vi "QX Thread.vi"() -> ()   [LabVIEW 2016]
uses:
  <vilib>/Utility/error.llb/DialogType.ctl
  Controls/hwSettings command.ctl
  DAQ-Display/Controls/PSDAQEG_Commoand Type.ctl
  DAQ-Display/PanelSplitToolkit/QueueManager.llb/CreatQueue.vi
  DAQ-Display/PanelSplitToolkit/QueueManager.llb/Remove.vi
  DAQ-Display/PanelSplitToolkit/QueueManager.llb/Insert.vi
  DAQ-Display/PanelSplitToolkit/QueueManager.llb/Destroy.vi
  DAQ-Display/PanelSplitToolkit/QueueManager.llb/Valid?.vi
panel:
  out "Waveform Chart":waveform(dbl)[](graph)
  out "Connect?":bool
  in  "Disconnect":bool
  in  "StopDAQ":bool
  in  "StartDAQ":bool
  in  "GetInfo":bool
  in  "Connect":bool
  in  "Caller":string
  # "QX硬件线程"
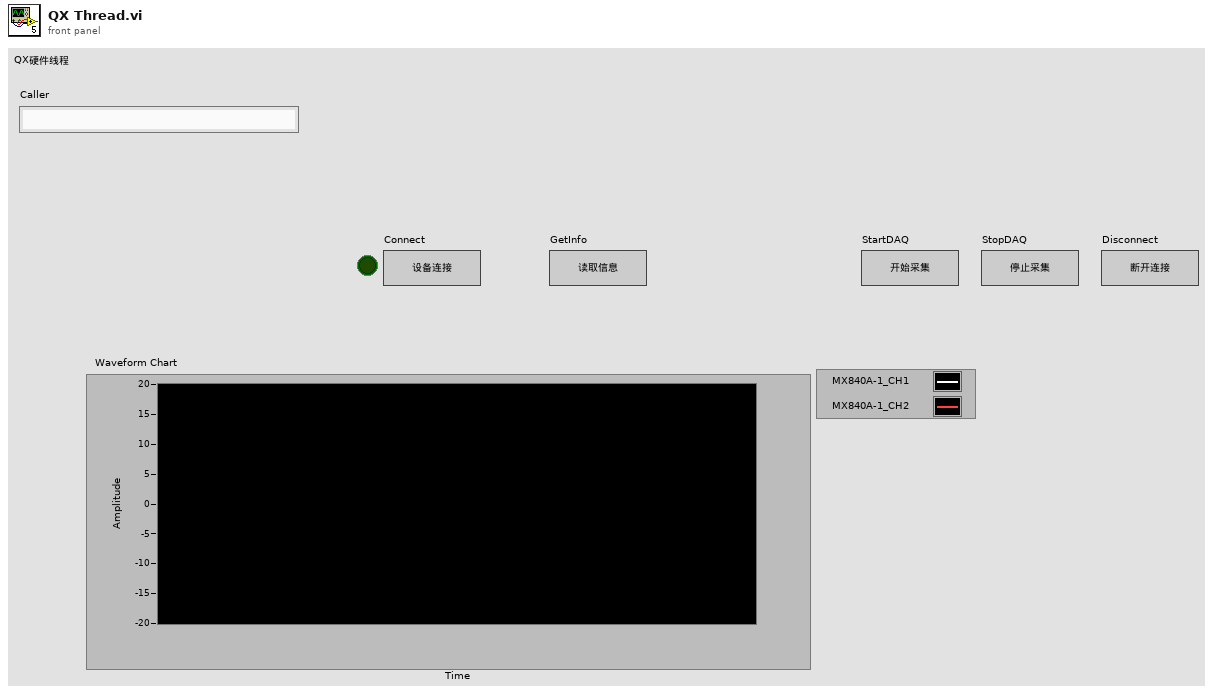
[diagram p1: front panel]
types:
  T1 = cluster{"Main Queue":string, "DAQ Queue":string, "ANA Queue":string, "CUI Queue":string, "Q-FocusList":string, "Q-Toolbar":string, "Q-Config":string}
  T2 = typedef "PSCHN_Channel Para.ctl" = cluster{"CHTag*":string, "Used?*":bool, "CHName":string, "Unit":string, "斜率":dbl, "截距":dbl}
  T3 = typedef "PSCHN_Card Para.ctl" = cluster{"Module Type":string, "Module Name":string, "ModuSN":string, "ModuIP":string, "Used?":bool, "Connected":bool, "Timing*":cluster{"Sample Rate":dbl}, "Channels":T2[]}
  T4 = typedef "hw_QX_hwDriverRef.ctl" = cluster{"DevicesAndSignals":cluster{"Devices":refnum<k24>[], "Signals":refnum<k24>[]}, "DaqMeasurement":refnum<k24>}
  T5 = cluster{"error":errorcluster, "LocalQ":cluster{"LQName":string, "LQEvent":string, "LQData":variant}, "HighQ":cluster{"HQName":string, "HQEvent":string, "HQData":variant}, "Channel":T2, "Card":T3, "hwType":string, "hwDriverRef":T4, "DevsInfo":T3[], "DataQ":string, "tdms ref":refnum<k34>, "Save":bool, "T0":timestamp}
  T6 = typedef "hwSettings command.ctl" = enum16{"Init", "Read", "Clear"}
  T7 = typedef "PSDAQEG_Commoand Type.ctl" = enum16{"Config", "Run", "Pause", "Stop", "Save", "Connect"}
  T8 = typedef "DialogType.ctl" = u16
  T9 = typedef "hwDefaultSetting.ctl" = cluster{"hwType":string, "hwNumber":u32, "hwName":string[], "hwSN":string[], "hwCHNumber":u32[]}
  T10 = cluster{string, string[], "Object Name":string}[]
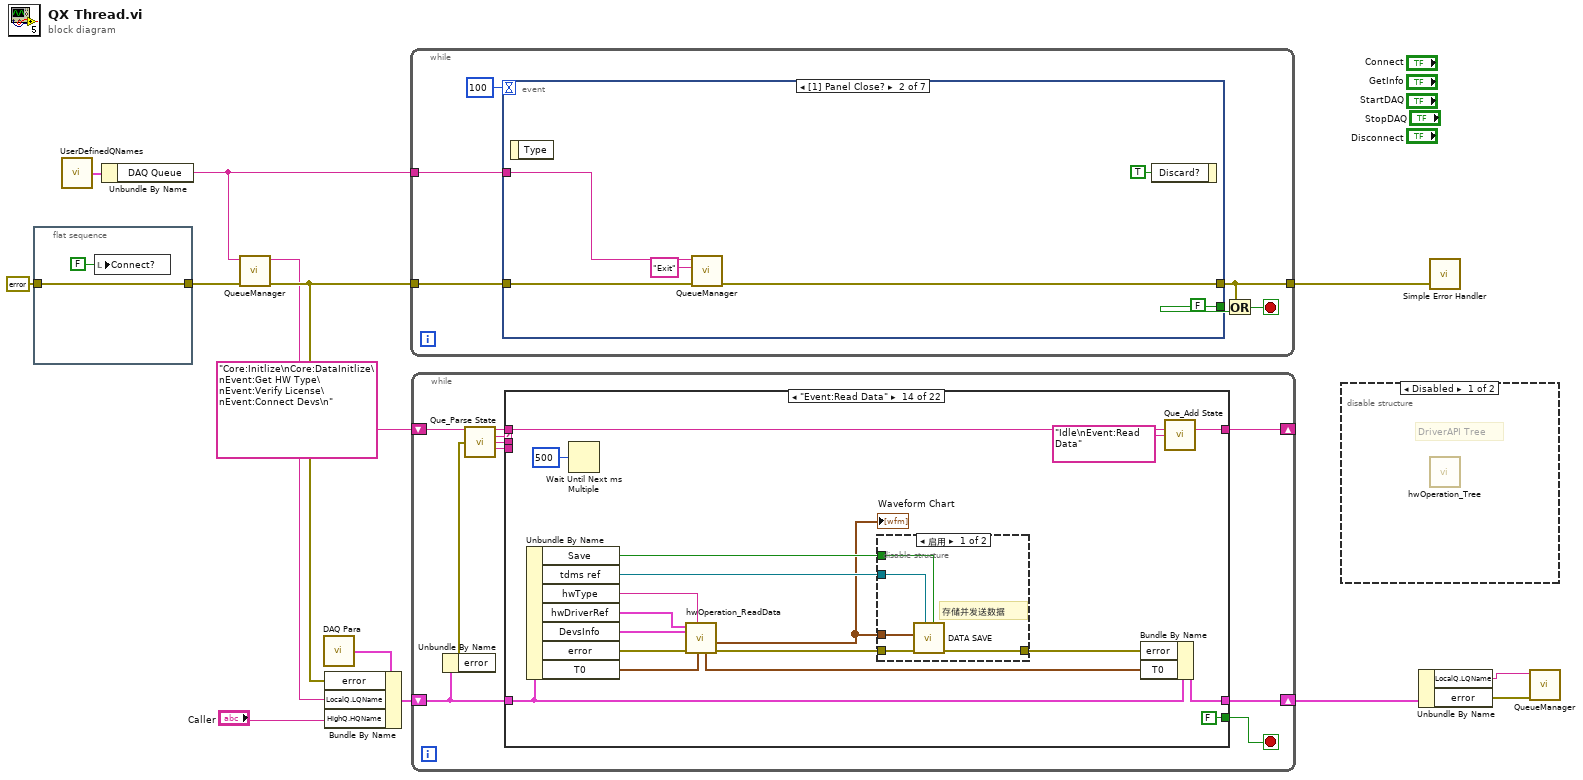
[diagram p0: block diagram]
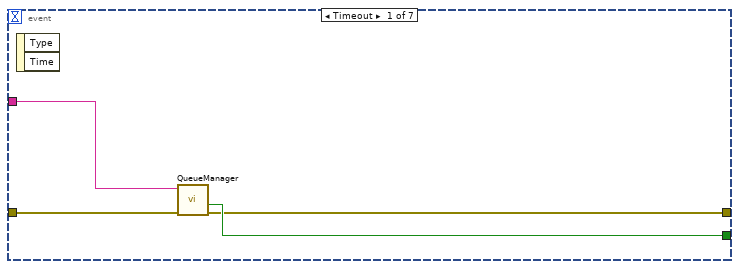
[diagram p3: hidden frame]
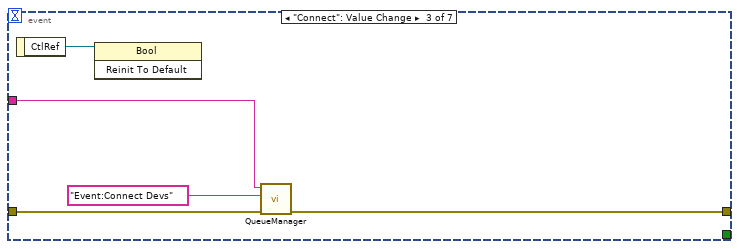
[diagram p4: hidden frame]
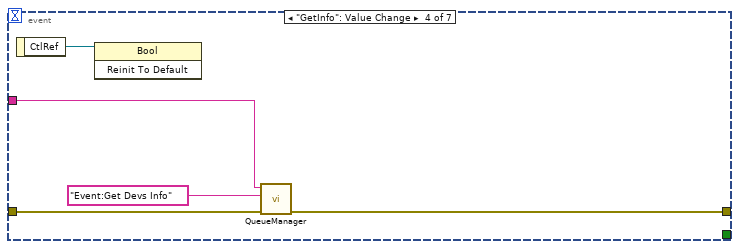
[diagram p5: hidden frame]
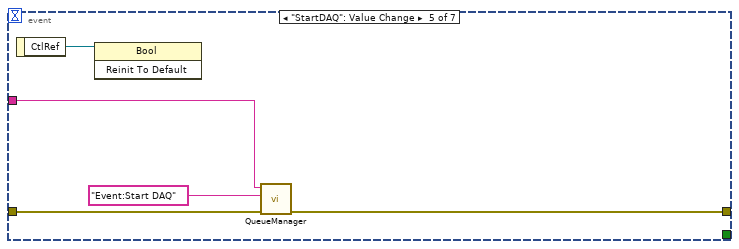
[diagram p6: hidden frame]
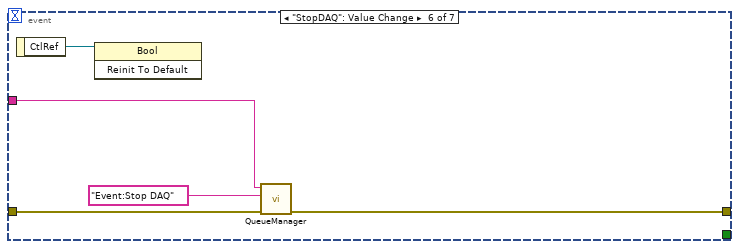
[diagram p7: hidden frame]
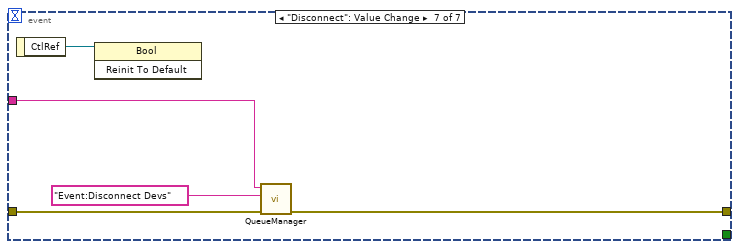
[diagram p8: hidden frame]
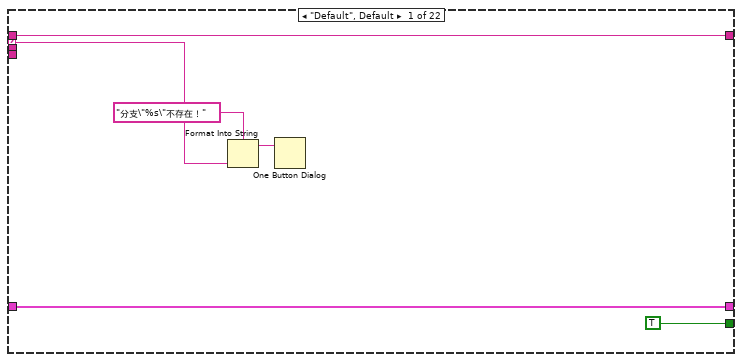
[diagram p9: hidden frame]
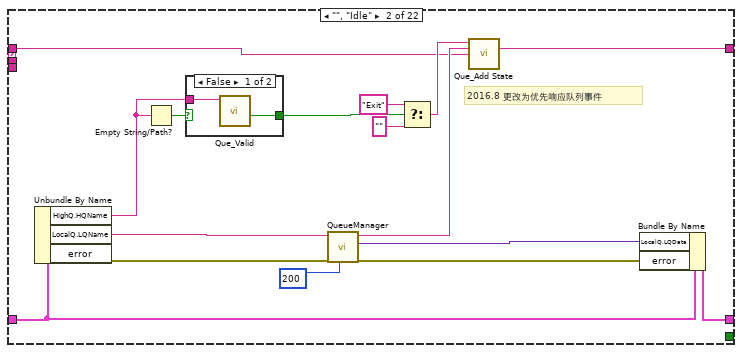
[diagram p10: hidden frame]
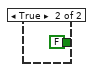
[diagram p11: hidden frame]
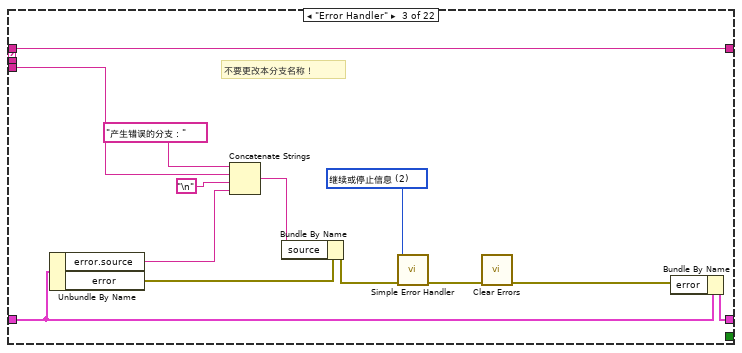
[diagram p12: hidden frame]
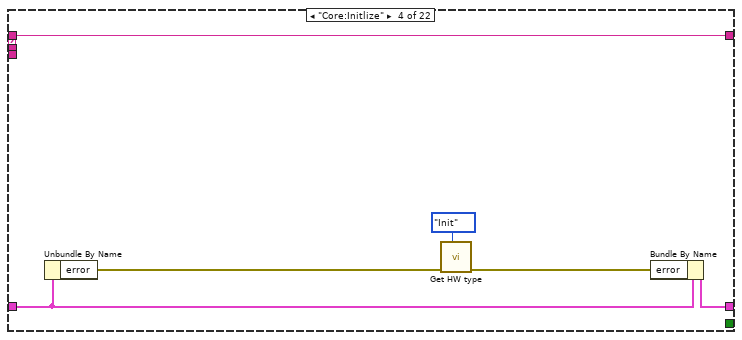
[diagram p13: hidden frame]
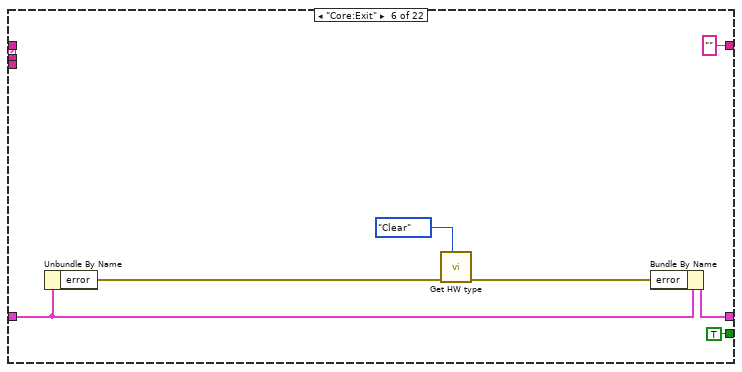
[diagram p15: hidden frame]
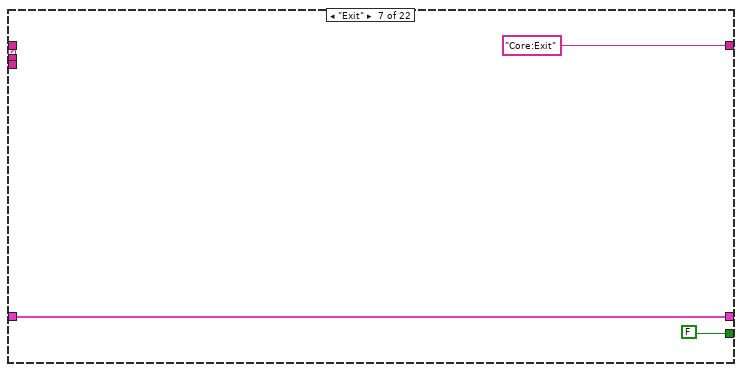
[diagram p16: hidden frame]
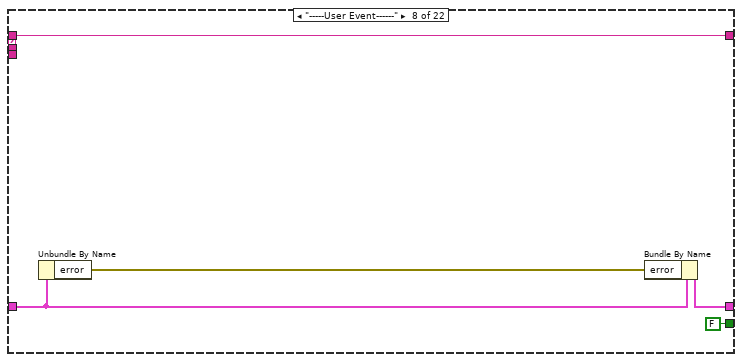
[diagram p17: hidden frame]
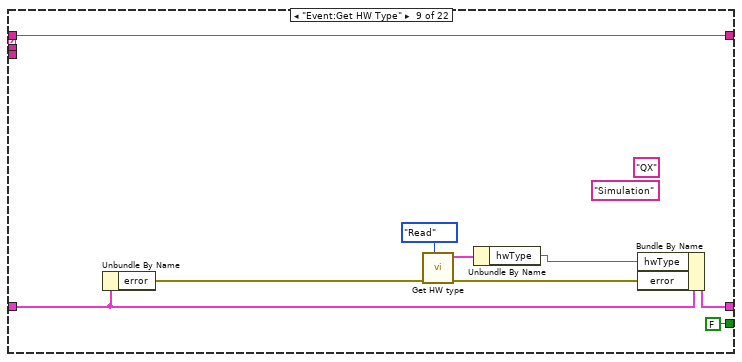
[diagram p18: hidden frame]
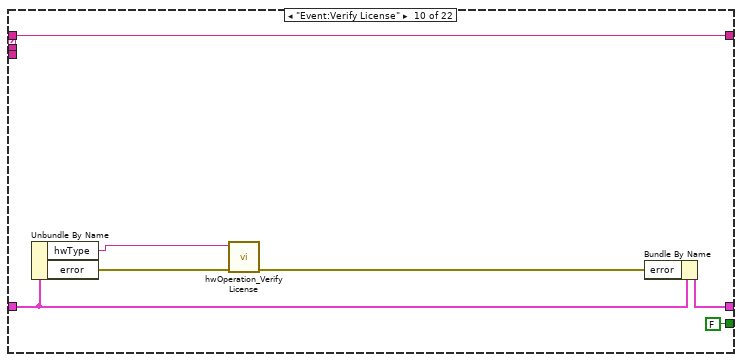
[diagram p19: hidden frame]
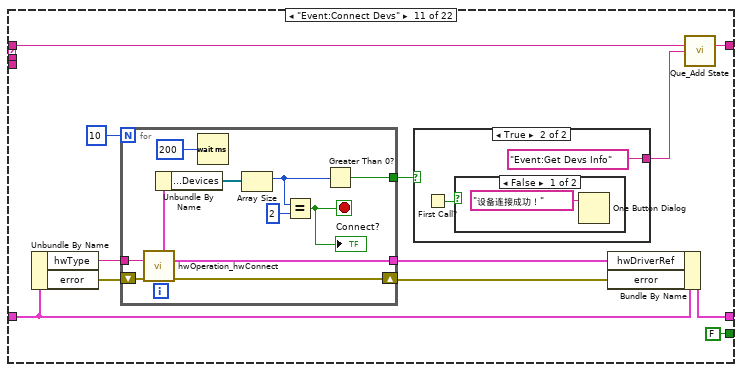
[diagram p20: hidden frame]
diagram:
  n1 = flat-sequence {
    tunnel: [w16] -> w3
    tunnel: errorcluster {"status"=FALSE, "code"=0, "source"=""} ("error in (no error)") -> [w16]
    frame #0 {
      n2 = local write "Connect?"(FALSE ("Connect?")) -> ()
    }
  }
  n3 = call "UserDefinedQNames.vi"() -> ("All Queues"=w1:T1)  [unwired: 11 in]
  n4 = Unbundle By Name(w1) -> ("DAQ Queue"=w9:string)
  n5 = call-poly "QueueManager.vi"("error in (no error)"=w3, "QueueName"=w9) -> ("error out"=w7:errorcluster, "QueueName out"=w6:string)  [unwired: 8 in]
  n6 = call "DAQ Para.vi"() -> ("Thread Para"=w4:T5)  [unwired: 2 in]
  n7 = Bundle By Name(cluster=w4, "error"=w7, "LocalQ.LQName"=w6, "HighQ.HQName"="Caller") -> (w10:T5)
  n8 = while {
    tunnel: w7 -> [w21]
    tunnel: w9 -> [w22]
    tunnel: [w18] -> w11
    stop <- w19 stop-if-true
    n9 = event shown="[1] Panel Close?" {
      selector: _ -> [_ _ _ _ _ _ _]
      dyn-events: _ -> [_ _ _ _ _ _ _]
      timeout: 100 -> [_ _ _ _ _ _ _]
      tunnel: [w24 FALSE _ _ _ _ _] -> w20
      tunnel: w22 -> [w26 w31 w34 w39 w44 w49 w54]
      tunnel: w21 -> [w25 w30 w35 w40 w45 w50 w55]
      tunnel: [w23 w29 w33 w38 w43 w48 w53] -> w18
      event Timeout {
        n10 = event-data() -> ()  [unwired: 1 in, 2 out]
        n11 = call-poly "QueueManager.vi"("error in (no error)"=w25, "Queue Name(unamed)"=w26) -> ("error out"=w23:errorcluster, "Not Exist?"=w24:bool)  [unwired: 8 in]
      }
      event Panel Close? {
        n12 = event-data() -> ()  [unwired: 1 in, 1 out]
        n13 = call-poly "QueueManager.vi"("error in"=w30, "Event"="Exit", "QueueName"=w31) -> ("error out"=w29:errorcluster)  [unwired: 7 in, 1 out]
        n14 = event-data("Discard?"=TRUE ("放弃？")) -> ()  [unwired: 1 in, 1 out]
      }
      event "Connect": Value Change {
        n15 = event-data() -> ("CtlRef"=w37:refnum<vi>)  [unwired: 1 in]
        n16 = invoke class="Bool" method="Reinit To Default"(reference=w37) -> ()  [unwired: 2 in, 3 out]
        n17 = call-poly "QueueManager.vi"("error in"=w35, "Event"="Event:Connect Devs", "QueueName"=w34) -> ("error out"=w33:errorcluster)  [unwired: 7 in, 1 out]
      }
      event "GetInfo": Value Change {
        n18 = event-data() -> ("CtlRef"=w42:refnum<vi>)  [unwired: 1 in]
        n19 = invoke class="Bool" method="Reinit To Default"(reference=w42) -> ()  [unwired: 2 in, 3 out]
        n20 = call-poly "QueueManager.vi"("error in"=w40, "Event"="Event:Get Devs Info", "QueueName"=w39) -> ("error out"=w38:errorcluster)  [unwired: 7 in, 1 out]
      }
      event "StartDAQ": Value Change {
        n21 = event-data() -> ("CtlRef"=w47:refnum<vi>)  [unwired: 1 in]
        n22 = invoke class="Bool" method="Reinit To Default"(reference=w47) -> ()  [unwired: 2 in, 3 out]
        n23 = call-poly "QueueManager.vi"("error in"=w45, "Event"="Event:Start DAQ", "QueueName"=w44) -> ("error out"=w43:errorcluster)  [unwired: 7 in, 1 out]
      }
      event "StopDAQ": Value Change {
        n24 = event-data() -> ("CtlRef"=w52:refnum<vi>)  [unwired: 1 in]
        n25 = invoke class="Bool" method="Reinit To Default"(reference=w52) -> ()  [unwired: 2 in, 3 out]
        n26 = call-poly "QueueManager.vi"("error in"=w50, "Event"="Event:Stop DAQ", "QueueName"=w49) -> ("error out"=w48:errorcluster)  [unwired: 7 in, 1 out]
      }
      event "Disconnect": Value Change {
        n27 = event-data() -> ("CtlRef"=w57:refnum<vi>)  [unwired: 1 in]
        n28 = invoke class="Bool" method="Reinit To Default"(reference=w57) -> ()  [unwired: 2 in, 3 out]
        n29 = call-poly "QueueManager.vi"("error in"=w55, "Event"="Event:Disconnect Devs", "QueueName"=w54) -> ("error out"=w53:errorcluster)  [unwired: 7 in, 1 out]
      }
    }
    n30 = Or(x=w18, y=w20) -> (x .or. y?=w19:bool)
  }
  n31 = while {
    shift-right: [w61] -> w12
    shift-left: w10 -> [w62]
    shift-right: [w60] -> _
    shift-left: "Core:Initlize\nCore:DataInitlize\nEvent:Get HW Type\nEvent:Verify License\nEvent:Connect Devs\n" -> [w67]
    stop <- w64 stop-if-true
    n32 = Unbundle By Name(w62) -> ("error"=w63:errorcluster)
    n33 = call "Que_Parse State.vi"("State Queue"=w67, "Error In (no error)"=w63) -> ("Remaining States"=w66:string, "Current State"=w65:string, "Arguments"=w59:string, "PreState"=w58:string)  [unwired: 10 in]
    n34 = case shown="\"Event:Read Data\"" w65 {
      selector: w65 -> [w71 _ _ _ _ _ _ _ _ _ _ _ _ _ _ _ _ _ _ _ _ _]
      tunnel: w66 -> [w72 w74 w105 w111 w112 _ _ w127 w136 w143 w148 w173 _ w204 _ w234 w236 w251 w267 w312 w330 w339]
      tunnel: w59 -> [_ _ _ _ _ _ _ _ _ _ _ _ _ _ _ _ _ _ _ _ _ _]
      tunnel: [TRUE _ _ _ _ TRUE FALSE FALSE FALSE FALSE FALSE FALSE FALSE FALSE FALSE FALSE _ _ _ _ _ _] -> w64
      tunnel: w62 -> [w73 w84 w102 w107 w113 w118 w122 w124 w133 w141 w154 w180 w191 w209 w224 w232 w237 w241 w258 w309 w321 w335]
      tunnel: [w73 w88 w101 w106 w113 w117 w122 w126 w135 w142 w155 w181 w192 w210 w225 w233 w237 w239 w261 w308 w320 w334] -> w61
      tunnel: [w72 w86 w105 w111 w112 "" ("Remaining States") "Core:Exit" ("Remaining States") w127 w136 w143 w147 w172 "Event:Read Data" ("Remaining States") w203 "" ("Remaining States") w234 w236 w251 w266 w312 w330 w339] -> w60
      tunnel: w58 -> [_ _ w99 _ _ _ _ _ _ _ _ _ _ _ _ _ _ _ _ _ _ _]
      frame "Default", Default {
        n35 = Format Into String(format string="分支\"%s\"不存在！" ("格式字符串"), w71) -> (resulting string=w70:string)  [unwired: 2 in, 1 out]
        n36 = One Button Dialog(message=w70) -> ()  [unwired: 1 in, 1 out]
      }
      frame "", "Idle" {
        # "2016.8 更改为优先响应队列事件"
        n37 = Unbundle By Name(w84) -> ("HighQ.HQName"=w78:string, "LocalQ.LQName"=w83:string, "error"=w82:errorcluster)
        n38 = Empty String/Path?(string/path=w78) -> (empty?=w81:bool)
        n39 = case shown="False" w81 {
          tunnel: [w91 FALSE ("Not Exist?")] -> w80
          tunnel: w78 -> [w90 _]
          frame False {
            n40 = call "Que_Valid.vi"("Queue Name(unamed)"=w90) -> ("Not Exist?"=w91:bool)  [unwired: 9 in, 1 out]
          }
          frame True {
          }
        }
        n41 = call-poly "QueueManager.vi"("Time out(-1)"=200, "error in (no error)"=w82, "Queue Name"=w83) -> ("error out"=w89:errorcluster, "Data"=w87:variant, "Event"=w75:string)  [unwired: 5 in, 1 out]
        n42 = Select(t="Exit" ("Event"), s=w80, f="") -> (s? t:f=w76:string)
        n43 = call "Que_Add State.vi"("State(s) in Front (\"\")"=w76, "State(s) in (\"\")"=w75, "State(s) at Back (\"\")"=w74) -> ("States Out"=w86:string)  [unwired: 12 in]
        n44 = Bundle By Name(cluster=w84, "LocalQ.LQData"=w87, "error"=w89) -> (w88:T5)
      }
      frame "Error Handler" {
        w100 = T8 2 items=["无对话框", "确定信息", "继续或停止信息", "确定信息＋警告", "继续/停止+警告"] ("type of dialog (OK msg:1)")
        # "不要更改本分支名称！"
        n45 = Unbundle By Name(w102) -> ("error.source"=w93:string, "error"=w95:errorcluster)
        n46 = Concatenate Strings("产生错误的分支：" ("字符串"), w99, "\n", w93) -> (w96:string)
        n47 = Bundle By Name(cluster=w95, "source"=w96) -> (w94:errorcluster)
        n48 = call <vilib>:"Simple Error Handler.vi"("type of dialog (OK msg:1)"=w100, "error in (no error)"=w94) -> ("error out"=w103:errorcluster)  [unwired: 3 in, 4 out]
        n49 = call <vilib>:"Clear Errors.vi"("error in (no error)"=w103) -> ("error out"=w104:errorcluster)  [unwired: 5 in, 1 out]
        n50 = Bundle By Name(cluster=w102, "error"=w104) -> (w101:T5)
      }
      frame "Core:Initlize" {
        n51 = Unbundle By Name(w107) -> ("error"=w109:errorcluster)
        n52 = call "Get HW type.vi"("Comm"=hwSettings_command."Init", "error in (no error)"=w109) -> ("error out"=w108:errorcluster)  [unwired: 8 in, 1 out]
        n53 = Bundle By Name(cluster=w107, "error"=w108) -> (w106:T5)
      }
      frame "Core:DataInitlize" {
      }
      frame "Core:Exit" {
        n54 = Unbundle By Name(w118) -> ("error"=w115:errorcluster)
        n55 = call "Get HW type.vi"("Comm"=hwSettings_command."Clear", "error in (no error)"=w115) -> ("error out"=w114:errorcluster)  [unwired: 8 in, 1 out]
        n56 = Bundle By Name(cluster=w118, "error"=w114) -> (w117:T5)
      }
      frame "Exit" {
      }
      frame "-----User Event------" {
        n57 = Unbundle By Name(w124) -> ("error"=w125:errorcluster)
        n58 = Bundle By Name(cluster=w124, "error"=w125) -> (w126:T5)
      }
      frame "Event:Get HW Type" {
        (unwired) "Simulation" ("value")
        (unwired) "QX" ("value")
        n59 = Unbundle By Name(w133) -> ("error"=w132:errorcluster)
        n60 = call "Get HW type.vi"("Comm"=hwSettings_command."Read", "error in (no error)"=w132) -> ("error out"=w131:errorcluster, "hwDefaultSetting"=w130:T9)  [unwired: 8 in]
        n61 = Unbundle By Name(w130) -> ("hwType"=w129:string)
        n62 = Bundle By Name(cluster=w133, "hwType"=w129, "error"=w131) -> (w135:T5)
      }
      frame "Event:Verify License" {
        n63 = Unbundle By Name(w141) -> ("hwType"=w138:string, "error"=w140:errorcluster)
        n64 = call "hwOperation_Verify License.vi"("hwType"=w138, "Error in"=w140) -> ("Error out"=w139:errorcluster)  [unwired: 8 in]
        n65 = Bundle By Name(cluster=w141, "error"=w139) -> (w142:T5)
      }
      frame "Event:Connect Devs" {
        n66 = Unbundle By Name(w154) -> ("hwType"=w153:string, "error"=w152:errorcluster)
        n67 = for {
          N: 10 -> [_]
          tunnel: w153 -> [w170]
          shift-right: [w168] -> w151
          shift-left: w152 -> [w169]
          tunnel: [w165] -> w149
          tunnel: [w162] -> w146
          stop <- w166 stop-if-true
          n68 = call "hwOperation_hwConnect.vi"("hwType"=w170, "error in (no error)"=w169) -> ("error out"=w168:errorcluster, "hwDriverRef"=w165:T4)  [unwired: 7 in, 1 out]
          n69 = Unbundle By Name(w165) -> ("DevicesAndSignals.Devices"=w164:refnum<k24>[])
          n70 = Wait (ms)(milliseconds to wait=u32 200) -> ()  [unwired: 1 out]
          n71 = Array Size(array=w164) -> (size(s)=w163:i32)
          n72 = Equal?(x=w163, y=2) -> (x = y?=w166:bool)
          "Connect?" <- w166
          n73 = Greater Than 0?(x=w163) -> (x > 0?=w162:bool)
        }
        n74 = case shown="True" w146 {
          tunnel: [_ "Event:Get Devs Info"] -> w145
          frame False {
            n75 = One Button Dialog(message="设备连接失败！" ("消息")) -> ()  [unwired: 1 in, 1 out]
          }
          frame True {
            n76 = First Call?() -> (First Call?: T/F=w158:bool)
            n77 = case shown="False" w158 {
              frame False {
                n78 = One Button Dialog(message="设备连接成功！" ("消息")) -> ()  [unwired: 1 in, 1 out]
              }
              frame True {
              }
            }
          }
        }
        n79 = Bundle By Name(cluster=w154, "hwDriverRef"=w149, "error"=w151) -> (w155:T5)
        n80 = call "Que_Add State.vi"("State(s) in (\"\")"=w148, "State(s) at Back (\"\")"=w145) -> ("States Out"=w147:string)  [unwired: 13 in]
      }
      frame "Event:Get Devs Info" {
        n81 = Unbundle By Name(w180) -> ("hwType"=w179:string, "hwDriverRef"=w178:T4, "error"=w177:errorcluster)
        n82 = call "hwOperation_Get Devs Info.vi"("hwType"=w179, "error in"=w177, "hwDriverRef in"=w178) -> ("error out"=w176:errorcluster, "Devs Info"=w174:T3[], "hwDriverRef out"=w175:T4)  [unwired: 6 in]
        n83 = Bundle By Name(cluster=w180, "hwDriverRef"=w175, "DevsInfo"=w174, "error"=w176) -> (w181:T5)
        n84 = call "Que_Add State.vi"("State(s) in (\"\")"=w173, "State(s) at Back (\"\")"="COM : Send DevsInfo" ("State(s) at Back (\"\")")) -> ("States Out"=w172:string)  [unwired: 13 in]
      }
      frame "Event:Start DAQ" {
        n85 = Unbundle By Name(w191) -> ("hwType"=w190:string, "DevsInfo"=w185:T3[], "error"=w189:errorcluster, "hwDriverRef"=w184:T4)
        n86 = call "hwOperation_Start DAQ.vi"("hwType"=w190, "error in"=w189, "Devs Info in"=w185, "hwDriverRef in"=w184) -> ("error out"=w188:errorcluster, "hwDriverRef out"=w186:T4)  [unwired: 5 in, 1 out]
        n87 = Get Date/Time In Seconds() -> (seconds since 1Jan1904=w183:timestamp)
        n88 = Bundle By Name(cluster=w191, "T0"=w183, "hwDriverRef"=w186, "error"=w188) -> (w192:T5)
      }
      frame "Event:Read Data" {
        n89 = Unbundle By Name(w209) -> ("Save"=w198:bool, "tdms ref"=w199:refnum<k34>, "hwType"=w206:string, "hwDriverRef"=w207:T4, "DevsInfo"=w205:T3[], "error"=w208:errorcluster, "T0"=w196:timestamp)
        n90 = Wait Until Next ms Multiple(millisecond multiple=u32 500 ("毫秒倍数")) -> ()  [unwired: 1 out]
        n91 = call "hwOperation_ReadData.vi"("t0"=w196, "hwType"=w206, "error in"=w208, "Devs Info in"=w205, "hwDriverRef in"=w207) -> ("error out"=w201:errorcluster, "Waveform[]"=w194:waveform(dbl)[], "t0"=w195:timestamp)  [unwired: 3 in, 1 out]
        "Waveform Chart" <- w194
        n92 = disable-structure shown="启用" {
          disable-tunnel: w201 -> [w216 w217]
          disable-tunnel: [w215 w217] -> w200
          disable-tunnel: w199 -> [w214 _]
          disable-tunnel: w198 -> [w213 _]
          disable-tunnel: w194 -> [w212 _]
          frame Enabled {
            # "存储并发送数据"
            n93 = call "DATA SAVE.vi"("save"=w213, "tdms ref"=w214, "error in"=w216, "Wave"=w212) -> ("error out"=w215:errorcluster)  [unwired: 7 in]
          }
          frame Disabled {
          }
        }
        n94 = Bundle By Name(cluster=w209, "error"=w200, "T0"=w195) -> (w210:T5)
        n95 = call "Que_Add State.vi"("State(s) in (\"\")"=w204, "State(s) at Back (\"\")"="Idle\nEvent:Read Data" ("State(s) at Back (\"\")")) -> ("States Out"=w203:string)  [unwired: 13 in]
      }
      frame "Event:Stop DAQ" {
        n96 = Unbundle By Name(w224) -> ("hwType"=w221:string, "hwDriverRef"=w222:T4, "error"=w223:errorcluster)
        n97 = call "hwOperation_Stop DAQ.vi"("hwType"=w221, "error in"=w223, "hwDriverRef in"=w222) -> ("error out"=w219:errorcluster)  [unwired: 7 in, 1 out]
        n98 = call <vilib>:"Clear Errors.vi"("error in (no error)"=w219) -> ("error out"=w218:errorcluster)  [unwired: 5 in, 1 out]
        n99 = Bundle By Name(cluster=w224, "error"=w218) -> (w225:T5)
      }
      frame "Event:Disconnect Devs" {
        n100 = Unbundle By Name(w232) -> ("hwType"=w229:string, "hwDriverRef"=w230:T4, "error"=w231:errorcluster)
        n101 = call "hwOperation_hwDisconnect.vi"("hwType"=w229, "error in"=w231, "hwDriverRef in"=w230) -> ("error out"=w228:errorcluster)  [unwired: 7 in, 1 out]
        n102 = call <vilib>:"Clear Errors.vi"("error in (no error)"=w228) -> ("error out"=w227:errorcluster)  [unwired: 5 in, 1 out]
        n103 = Bundle By Name(cluster=w232, "error"=w227) -> (w233:T5)
      }
      frame "---与其它线程接口---" {
      }
      frame "Initlize DataQ" {
        w243 = "Analog CHs"
        # "不用每次初始化这个队列"
        n104 = Unbundle By Name(w241) -> ("DevsInfo"=w250:T3[], "error"=w242:errorcluster)
        n105 = for {
          tunnel: [w256] -> w249 mode=concatenating
          tunnel: w250 -> [w255] mode=indexing
          n106 = Unbundle By Name(w255) -> ("Channels"=w256:T2[])
        }
        n107 = for {
          tunnel: w249 -> [w254] mode=indexing
          tunnel: [w253] -> w248 mode=indexing if=w252
          n108 = Unbundle By Name(w254) -> ("CHTag*"=w253:string, "Used?*"=w252:bool)
        }
        n109 = Bundle(w243, w248, "Object Name"="Queue Type") -> (w246:cluster{string, string[], "Object Name":string})  [unwired: 1 in]
        n110 = Build Array(w246) -> (w245:T10)
        n111 = call "DAQEG_DAQ DATA Queue FGV.vi"("Command"=enum16{"Initialize", "Get Value", "Set Value"}."Set Value", "error in (no error)"=w242, "DAQ DATA"=w245) -> ("error out"=w244:errorcluster)  [unwired: 7 in, 1 out]
        n112 = call "PSDS_Create Object.vi"("error in (no error)"=w244, "Object Name"=w243) -> ("error out"=w240:errorcluster)  [unwired: 8 in, 1 out]
        n113 = Bundle By Name(cluster=w241, "error"=w240) -> (w239:T5)
      }
      frame "COM : DAQ_CMD" {
        # "接收开始、停止等按钮的信息，跳转到相应的分支"
        n114 = Unbundle By Name(w258) -> ("LocalQ.LQData"=w269:variant, "error"=w270:errorcluster)
        n115 = Variant To Data(error in=w270, type=cluster{"Command":T7, "Data":variant} {"Command"=enum."Run", "Data"=variant} ("输出簇"), Variant=w269) -> (data=w265:cluster{"Command":T7, "Data":variant}, error out=w264:errorcluster)
        n116 = Unbundle By Name(w265) -> ("Command"=w263:T7, "Data"=w262:variant)
        n117 = case shown="\"Save\"" w263 {
          tunnel: w264 -> [w272 w281 w283 w289 w293 w298]
          tunnel: w262 -> [_ w280 _ _ _ w296]
          tunnel: [w272 w278 w283 w289 w293 w297] -> w260
          tunnel: ["" "Initlize DataQ\nEvent:Start DAQ" "" "Event:Stop DAQ" "Event:Connect Devs" ""] -> w259
          tunnel: w258 -> [w271 w276 w282 w288 w292 w301]
          tunnel: [w271 w275 w282 w287 w292 w300] -> w257
          frame "Config", Default {
            # "暂未用到"
          }
          frame "Run" {
            n118 = Variant To Data(error in=w281, type=timestamp(0 s since 1904-01-01) ("当前时间"), Variant=w280) -> (data=w274:timestamp, error out=w278:errorcluster)
            n119 = Bundle By Name(cluster=w276, "T0"=w274) -> (w275:T5)
          }
          frame "Pause" {
            # "暂不添加功能"
          }
          frame "Stop" {
            n120 = Bundle By Name(cluster=w288, "tdms ref"=refnum<k34> refnum, "Save"=FALSE) -> (w287:T5)
          }
          frame "Connect" {
          }
          frame "Save" {
            n121 = Variant To Data(error in=w298, type=refnum<k34> refnum ("tdms ref"), Variant=w296) -> (data=w294:refnum<k34>, error out=w297:errorcluster)
            n122 = Bundle By Name(cluster=w301, "tdms ref"=w294, "Save"=TRUE) -> (w300:T5)
          }
        }
        n123 = Bundle By Name(cluster=w257, "error"=w260) -> (w261:T5)
        n124 = call "Que_Add State.vi"("State(s) in (\"\")"=w267, "State(s) at Back (\"\")"=w259) -> ("States Out"=w266:string)  [unwired: 13 in]
      }
      frame "COM : DAQ_CFG Updata" {
        # "只接收已连接的卡信息"
        # "接收配置UI线程发来的配置信息"
        n125 = Unbundle By Name(w309) -> ("DevsInfo"=w306:T3[], "LocalQ.LQData"=w310:variant, "error"=w311:errorcluster)
        n126 = Variant To Data(error in=w311, type=w306, Variant=w310) -> (data=w305:T3[], error out=w307:errorcluster)
        n127 = for {
          tunnel: w306 -> [w319] mode=indexing
          tunnel: [w318] -> w304 mode=indexing
          n128 = Unbundle By Name(w319) -> ("ModuSN"=w318:string)
        }
        n129 = for {
          tunnel: w305 -> [w314] mode=indexing
          tunnel: w304 -> [w317]
          tunnel: [w314] -> w303 mode=indexing if=w313
          n130 = Unbundle By Name(w314) -> ("ModuSN"=w316:string)
          n131 = Search 1D Array(1D array=w317, element=w316) -> (index of element=w315:i32)  [unwired: 1 in]
          n132 = Greater Or Equal To 0?(x=w315) -> (x >= 0?=w313:bool)
        }
        n133 = Bundle By Name(cluster=w309, "DevsInfo"=w303, "error"=w307) -> (w308:T5)
      }
      frame "COM : Request DevsInfo" {
        # "这个常量没有用"
        # "发送DeviceInfo至发出请求的队列"
        n134 = Unbundle By Name(w321) -> ("DevsInfo"=w326:T3[], "LocalQ.LQData"=w329:variant, "error"=w328:errorcluster)
        n135 = call <vilib>:"Space Constant.vi"() -> ("String"=w324:string)
        n136 = Variant To Data(error in=w328, type=w324, Variant=w329) -> (data=w325:string, error out=w327:errorcluster)
        n137 = call-poly "QueueManager.vi"("error in"=w327, "Data"=w326, "Event"="data", "QueueName"=w325) -> ("error out"=w322:errorcluster)  [unwired: 6 in, 1 out]
        n138 = Bundle By Name(cluster=w321, "error"=w322) -> (w320:T5)
      }
      frame "COM : Send DevsInfo" {
        # "连接成功后主动向配置线程发送DevsInfo。\n配置线程将会用到里面的Module Name、Module IP、CHTag[]等信息。"
        n139 = Unbundle By Name(w335) -> ("DevsInfo"=w338:T3[], "error"=w333:errorcluster)
        n140 = call "UserDefinedQNames.vi"() -> ("All Queues"=w332:T1)  [unwired: 11 in]
        n141 = Unbundle By Name(w332) -> ("Q-Config"=w331:string)
        n142 = call-poly "QueueManager.vi"("error in"=w333, "Data"=w338, "Event"="COM : Receive DevsInfo", "QueueName"=w331) -> ("error out"=w336:errorcluster)  [unwired: 6 in, 1 out]
        n143 = Bundle By Name(cluster=w335, "error"=w336) -> (w334:T5)
      }
    }
  }
  n144 = disable-structure shown="Disabled" {
    frame Disabled {
      # "DriverAPI Tree"
      n145 = call "hwOperation_Tree.vi"() -> ()  [unwired: 12 in]
    }
    frame Enabled {
    }
  }
  n146 = Unbundle By Name(w12) -> ("LocalQ.LQName"=w8:string, "error"=w13:errorcluster)
  n147 = call <vilib>:"Simple Error Handler.vi"("error in (no error)"=w11) -> ()  [unwired: 4 in, 5 out]
  n148 = call-poly "QueueManager.vi"("error in (no error)"=w13, "QueeuName"=w8) -> ()  [unwired: 9 in, 1 out]
